vi "PCO_GetInfoString.vi"(8 "error in (no error)":errorcluster {"code" format="%x"}, 10 "dwinfotype":u32, 11 "ph":u64) -> (0 "error out":errorcluster {"code" format="%x"}, 1 "infoString":string, 2 "ErrorMessage":i32 format="%x", 3 "ph out":u64)   [LabVIEW 2020, in "SDK.lvlib" / "GeneralCameraStatus.lvlib"]
doc: "<b>Description:</b>\nThis function retrieves some information about the camera, e.g. sensor name. A zero terminated ASCII string will be returned in the provided array. This array must be large enough to hold the complete string and the termination value, if not, an error will be returned. At most 500 bytes will be returned from the camera. If a specific info type is not available for the camera an error will be returned.\n\n<b>Supported camera type:</b>\nAll cameras\n\n<b>Descriptor dependency:</b>\nNone"
uses:
  GeneralCameraStatus.lvlib
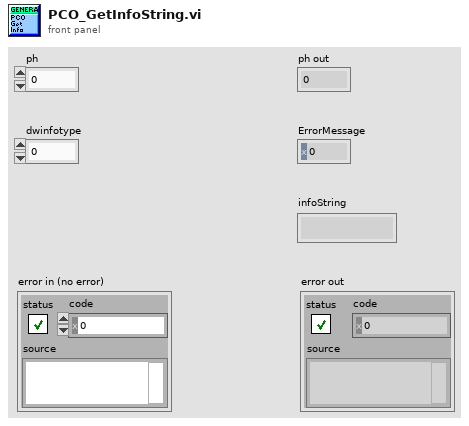
[diagram p1: front panel]
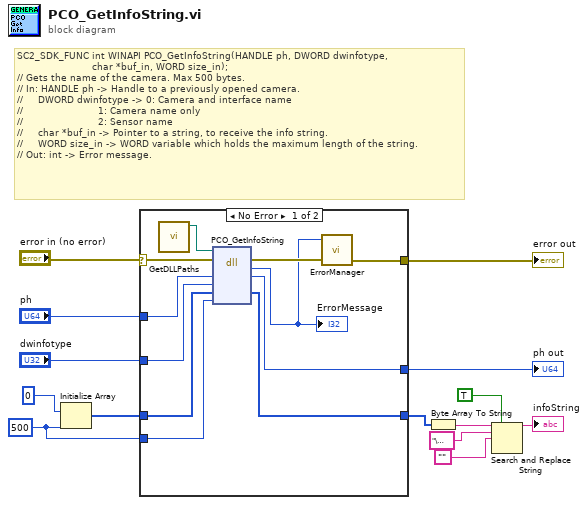
[diagram p0: block diagram]
diagram:
  w8 = u16 500 ("dimension size")
  # "SC2_SDK_FUNC int WINAPI PCO_GetInfoString(HANDLE ph, DWORD dwinfotype,\n                         char *buf_in, WORD size_in);\n// Gets the name of the camera. Max 500 bytes.\n// In: HANDLE ph -> Handle to a previously opened camera.\n//     DWORD dwinfotype -> 0: Camera and interface name\n//                         1: Camera name only\n//                         2: Sensor name\n//     char *buf_in -> Pointer to a string, to receive the info string.\n//     WORD size_in -> WORD variable which holds the maximum length of the string.\n// Out: int -> Error message."
  n1 = Initialize Array(u8 0 ("element"), w8) -> (w7:u8[])
  n2 = case shown="No Error" "error in (no error)" {
    selector: "error in (no error)" -> [w20 w28]
    tunnel: "ph" -> [w25 w27]
    tunnel: [w24 w27] -> w13
    tunnel: [w22 w28] -> w12
    tunnel: "dwinfotype" -> [w19 _]
    tunnel: w8 -> [w18 _]
    tunnel: w7 -> [w17 w26]
    tunnel: [w16 w26] -> w2
    frame No Error {
      n3 = call "GetDLLPaths.vi"() -> ("SC2_Cam_Path"=w15:path)  [unwired: 9 in, 2 out]
      n4 = dll-call lib="?" fn="PCO_GetInfoString"(path in=w15, error in=w20, "ph"=w25, "dwinfotype"=w19, "buf_in"=w17, "size_in"=w18) -> (error out=w23:errorcluster, "return type"=w21:i32, "ph"=w24:u64, "buf_in"=w16:u8[])  [unwired: 3 in, 1 out]
      "ErrorMessage" <- w21
      n5 = call "ErrorManager.vi"("error in (no error)"=w23, "error code"=w21) -> ("error out"=w22:errorcluster)  [unwired: 3 in]
    }
    frame Error {
    }
  }
  "ph out" <- w13
  "error out" <- w12
  n6 = Byte Array To String(unsigned byte array=w2) -> (string=w6:string)
  n7 = Search and Replace String(replace all?=TRUE ("replace all? (F)"), input string=w6, search string="\u0000", replace string="" ("replace string (\"\")")) -> (result string=→"infoString":string)  [unwired: 4 in, 3 out]
